vi "TestDialogObserve_RequestDblX_XPublished_ValueReceived.vi"(8 "error in (no error)":errorcluster, 11 "TestCase in":refnum<class "TestDialogBox.lvclass">) -> (0 "error out":errorcluster, 3 "TestCase out":refnum<class "TestDialogBox.lvclass">)   [LabVIEW 2018, in "TestDialogBox.lvclass"]
uses:
  TestDialogBox.lvclass
  Doubles/ModelPublishesDblX/ModelPublishesDblX.lvclass
  modules/mva-viewable/Source/IViewModel/IViewModel/IViewModel.lvclass
  C:/Program Files (x86)/National Instruments/LabVIEW 2018/vi.lib/ActorFramework/Actor/Actor.lvclass
  modules/mva-core/Source/Mediator/Mediator/Mediator.lvclass
  Doubles/DialogBoxSubscribesToDblX/DialogBoxSubscribesToDblX.lvclass/DialogBoxSubscribesToDblX.ctl
  Doubles/ViewableLaunchesDialogBox/ViewableLaunchesDialogBox.lvclass/ViewableLaunchesDialogBox.ctl
  modules/composed-event-logger/Source/Composed Log/LoggerReference/LoggerReference.lvclass/LoggerReference.ctl
  modules/mva-core/Source/IObserver/IObserver/IObserver.lvclass/IObserver.ctl
  modules/mva-core/Source/IMediator/IMediator/IMediator.lvclass/IMediator.ctl
  modules/mva-viewable/Source/IViewModel/IViewModel/IViewModel.lvclass/IViewModel.ctl
  modules/mva-viewable/Source/IViewManager/IViewManager Messages/Launch Nested Views Msg/Launch Nested Views Msg.lvclass/Launch Nested Views Msg.ctl
  modules/mva-viewable/Source/IViewManager/IViewManager/IViewManager.lvclass/IViewManager.ctl
  <vilib>/ActorFramework/Message Enqueuer/Message Enqueuer.lvclass/Message Enqueuer.ctl
  a0531555-97ce-47e1-90de-d612bf905464.vi
  a0531555-97ce-47e1-90de-d612bf905464.vi/4b58e03c-be92-4cd2-9125-f78d078cfd67.vi
  modules/mva-core/Source/IObserver/IObserver/Configure Observer Logging.vi
  modules/mva-viewable/Source/IViewModel/IViewModel/Write Startup Model-View Configuration.vi
  modules/mva-core/Source/IMediator/IMediator/Configure Mediator.vi
  <vilib>/ActorFramework/Message Enqueuer/Enqueue.vi
  modules/composed-event-logger/Source/Composed Log/LoggerReference/Return Aggregate Queues.vi
  modules/composed-event-logger/Source/Composed Log/LoggerReference/Add Aggregate Log.vi
  a0531555-97ce-47e1-90de-d612bf905464.vi/4b58e03c-be92-4cd2-9125-f78d078cfd67.vi/467b9aba-ab44-4297-978f-72bf0771973b.vi
  modules/mva-viewable/Source/IViewManager/IViewManager Messages/Launch Nested Views Msg/Pack Launch Nested Views Msg.vi
  modules/mva-viewable/Source/IViewManager/IViewManager/Write Startup Launch Nested Views Msg.vi
  modules/composed-event-logger/Source/Composed Log/LoggerReference/Send Add Sink.vi
  Doubles/DialogBoxSubscribesToDblX/DialogBoxSubscribesToDblX.lvclass
  modules/composed-event-logger/Source/Text File Sink/Text File Sink.lvclass
  Doubles/ViewableLaunchesDialogBox/ViewableLaunchesDialogBox.lvclass
  <vilib>/ActorFramework/Stop Msg/Stop Msg.lvclass
  C:/Program Files (x86)/National Instruments/LabVIEW 2018/vi.lib/ActorFramework/Message/Message.lvclass
  modules/composed-event-logger/Source/Composed Log/Application Logger/Launch Worker Loop.vi
  modules/composed-event-logger/Source/Composed Log/LoggerReference/Initialize Logger Instance.vi
  <vilib>/ActorFramework/Message Priority Queue/Priority Enqueue.vi
  modules/mva-viewable/Source/IViewable/IApplicationStyle/IApplicationStyle.lvclass
  modules/composed-event-logger/Source/Composed Log/LoggerReference/LoggerReference.lvclass
  modules/composed-event-logger/Source/Composed Log/IErrorFormat/IErrorFormat.lvclass
  modules/composed-event-logger/Source/Composed Log/Log Sink/Log Sink.lvclass
  modules/mva-viewable/Source/IViewManager/IViewManager Messages/Launch Nested Views Msg/Launch Nested Views Msg.lvclass
  <vilib>/ActorFramework/Actor/Actor.lvclass
panel:
  out "Dialog Observation":cluster{dbl, "error constant":errorcluster}
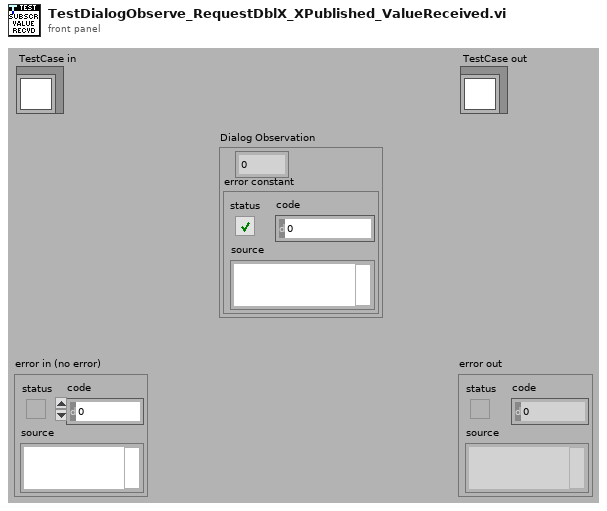
[diagram p1: front panel]
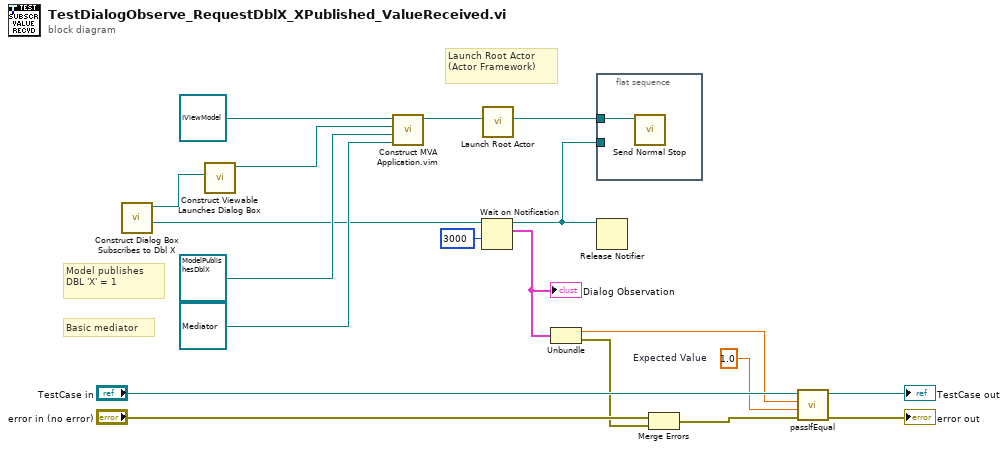
[diagram p0: block diagram]
diagram:
  w3 = 1.0  # Expected Value
  # "Model publishes\nDBL 'X' = 1"
  # "Basic mediator"
  # "Launch Root Actor\n(Actor Framework)"
  n1 = call "Construct Dialog Box Subscribes to Dbl X.vi"() -> ("Datum Received Notifier"=w9:refnum<notifier>, "DialogBoxSubscribesToDblX"=w10:refnum<class "DialogBoxSubscribesToDblX.lvclass">)  [unwired: 10 in]
  n2 = call "Construct Viewable Launches Dialog Box.vi"("DialogBox to Launch"=w10) -> ("ViewableLaunchesDialogBox"=w11:refnum<class "ViewableLaunchesDialogBox.lvclass">)  [unwired: 10 in]
  n3 = call "Construct MVA Application.vim"("Mediator Type"=refnum<class "Mediator.lvclass"> refnum ("Mediator.lvlib:Mediator.lvclass"), "Model Type"=refnum<class "ModelPublishesDblX.lvclass"> refnum ("ModelPublishesDblX.lvclass"), "Startup View Configuration"=w11, "IViewModel In"=refnum<class "IViewModel.lvclass"> refnum ("IViewModel.lvlib:IViewModel.lvclass")) -> ("IViewModel Out"=w13:refnum<class "IViewModel.lvclass">)  [unwired: 7 in]
  n4 = Wait on Notification(notifier=w9, timeout in ms (-1)=3000) -> (notifier out=w1:refnum<notifier>, notification=w7:cluster{dbl, "error constant":errorcluster})  [unwired: 2 in, 2 out]
  "Dialog Observation" <- w7
  n5 = call <vilib>:"Launch Root Actor.vi"("Actor"=w13) -> ("Actor's Enqueuer"=w2:refnum<class "Message Enqueuer.lvclass">)  [unwired: 9 in, 1 out]
  n6 = Unbundle(w7) -> (w4:dbl, "error constant"=w5:errorcluster)
  n7 = flat-sequence {
    tunnel: w2 -> [w20]
    tunnel: w1 -> [_]
    frame #0 {
      n8 = call <vilib>:"Send Normal Stop.vi"("Message Enqueuer"=w20) -> ()  [unwired: 10 in, 1 out]
    }
  }
  n9 = Release Notifier(notifier=w1) -> ()  [unwired: 2 in, 3 out]
  n10 = Merge Errors("error in (no error)", w5) -> (w6:errorcluster)
  n11 = call-dynamic "passIfEqual.vi"("error in (no error)"=w6, "y"=w3, "x"=w4, "TestCase in"="TestCase in") -> ("error out"=→"error out":errorcluster, "TestCase out"=→"TestCase out":refnum<class "TestDialogBox.lvclass">)  [unwired: 6 in]
